vi "Cmd1.vi"(8 "error in (no error)":errorcluster, 11 "VISA Refnum in":refnum<visa-resource-name>) -> (0 "error out (no error)":errorcluster, 1 "read buffer":string, 3 "VISA Refnum in 2":refnum<visa-resource-name>, 4 "Señales Digitales":dynamicdata(graph), 6 "Señales Analógicas":dynamicdata(graph), 7 "Señales":T1)   [LabVIEW 2020]
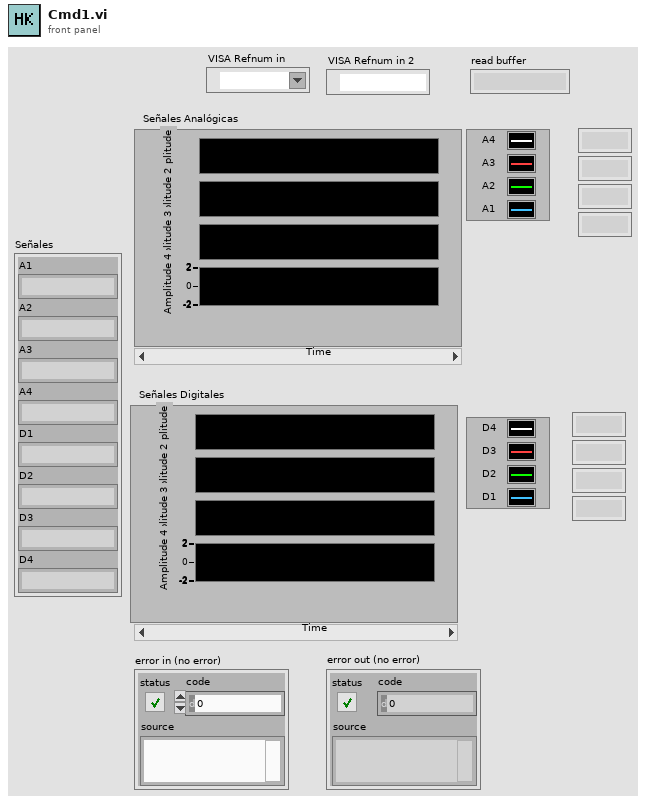
[diagram p1: front panel]
types:
  T1 = cluster{"A1":string, "A2":string, "A3":string, "A4":string, "D1":string, "D2":string, "D3":string, "D4":string}
  T2 = cluster{"[0]":string, "[1]":string, "[2]":string, "[3]":string, "[4]":string, "[5]":string, "[6]":string, "[7]":string, "[8]":string}
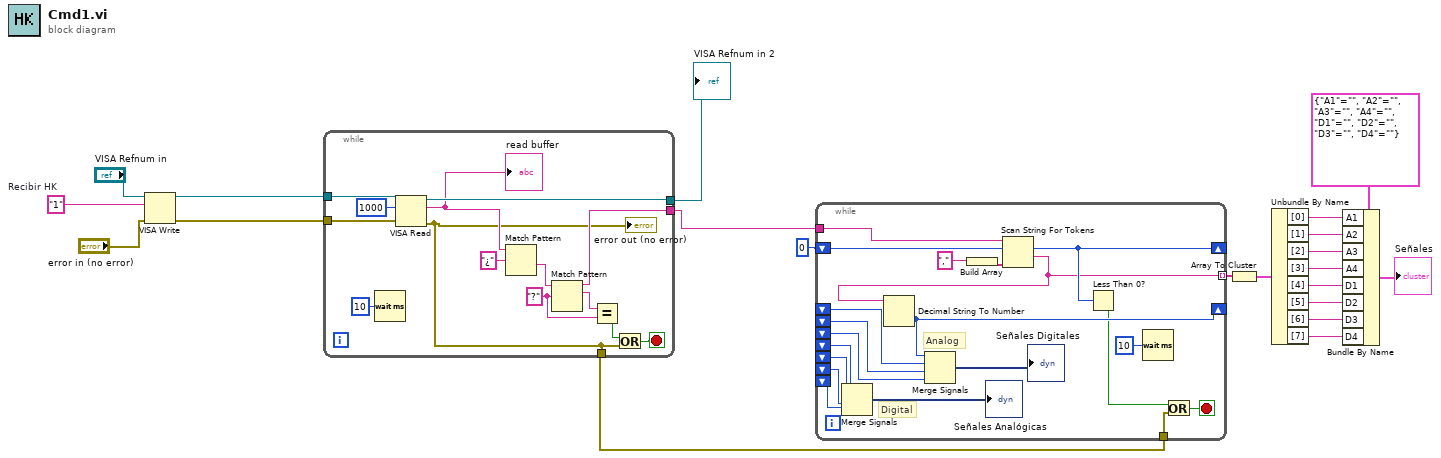
[diagram p0: block diagram]
diagram:
  w21 = "1"  # Recibir HK
  n1 = VISA Write(VISA resource name="VISA Refnum in", write buffer=w21, error in (no error)="error in (no error)") -> (VISA resource name out=w17:refnum<visa-resource-name>, error out=w16:errorcluster)  [unwired: 1 out]
  n2 = while {
    tunnel: w17 -> [w35]
    tunnel: w16 -> [w34]
    tunnel: [w31] -> w3
    tunnel: [w25] -> w2
    tunnel: [w22] -> w1
    stop <- w26 stop-if-true
    w28 = "?" ("regular expression")
    n3 = Wait (ms)(milliseconds to wait=u32 10) -> ()  [unwired: 1 out]
    n4 = VISA Read(VISA resource name=w35, byte count=u32 1000, error in (no error)=w34) -> (VISA resource name out=w25:refnum<visa-resource-name>, read buffer=w23:string, error out=w22:errorcluster)  [unwired: 1 out]
    "error out (no error)" <- w22
    "read buffer" <- w23
    n5 = Match Pattern(string=w23, regular expression="¿") -> (after substring=w32:string)  [unwired: 1 in, 3 out]
    n6 = Match Pattern(string=w32, regular expression=w28) -> (before substring=w31:string, match substring=w29:string)  [unwired: 1 in, 2 out]
    n7 = Equal?(x=w29, y=w28) -> (x = y?=w27:bool)
    n8 = Or(x=w27, y=w22) -> (x .or. y?=w26:bool)
  }
  "VISA Refnum in 2" <- w2
  n9 = while {
    shift-right: [w52] -> _
    shift-left: 0 -> [w53]
    tunnel: [w50] -> w7 mode=indexing
    tunnel: w3 -> [w51]
    shift-right: [w42] -> _
    shift-left: _ -> [w43]
    shift-left: _ -> [w44]
    shift-left: _ -> [w45]
    shift-left: _ -> [w46]
    shift-left: _ -> [w47]
    shift-left: _ -> [w48]
    shift-left: _ -> [w49]
    tunnel: w1 -> [w36]
    stop <- w38 stop-if-true
    # "Digital"
    # "Analog"
    n10 = Merge Signals(w46, w47, w48, w49) -> (→"Señales Analógicas":dynamicdata)
    n11 = Build Array("," ("search string/char (-)")) -> (w54:string[])
    n12 = Scan String For Tokens(6:w54, 8:w53, 9:w51) -> (1:w50:string, 2:w52:i32)  [unwired: 3 in, 2 out]
    n13 = Decimal String To Number(string=w50) -> (number=w42:i32)  [unwired: 2 in, 1 out]
    n14 = Merge Signals(w42, w43, w44, w45) -> (→"Señales Digitales":dynamicdata)
    n15 = Less Than 0?(x=w52) -> (x < 0?=w37:bool)
    n16 = Wait (ms)(milliseconds to wait=u32 10) -> ()  [unwired: 1 out]
    n17 = Or(x=w37, y=w36) -> (x .or. y?=w38:bool)
  }
  n18 = Array To Cluster(array=w7) -> (cluster=w15:T2)
  n19 = Unbundle By Name(w15) -> ("[0]"=w9:string, "[1]"=w14:string, "[2]"=w13:string, "[3]"=w12:string, "[4]"=w11:string, "[5]"=w4:string, "[6]"=w5:string, "[7]"=w6:string)
  n20 = Bundle By Name(cluster=T1 {"A1"="", "A2"="", "A3"="", "A4"="", "D1"="", "D2"="", "D3"="", "D4"=""}, "A1"=w9, "A2"=w14, "A3"=w13, "A4"=w12, "D1"=w11, "D2"=w4, "D3"=w5, "D4"=w6) -> (→"Señales":T1)
